vi "Stop.vi"(8 "Error In":errorcluster, 11 "object in":refnum<class "OWON SDS1022.lvclass">) -> (0 "Error Out":errorcluster, 3 "object out":refnum<class "OWON SDS1022.lvclass">)   [LabVIEW 2023, in "OWON SDS1022.lvlib" / "OWON SDS1022.lvclass"]
uses:
  OWON SDS1022.lvclass
  OWON SDS1022.lvclass/OWON SDS1022.ctl
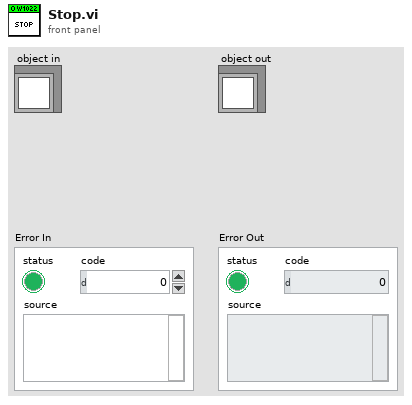
[diagram p1: front panel]
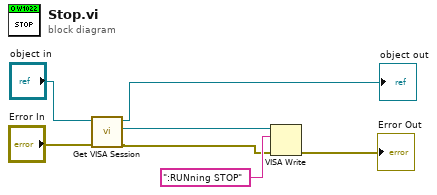
[diagram p0: block diagram]
diagram:
  n1 = call-dynamic "Get VISA Session.vi"("error in"="Error In", "Scope VISA in"="object in") -> ("error out"=w1:errorcluster, "VISA session"=w7:refnum<visa-resource-name>, "Scope VISA out"=→"object out":refnum<class "OWON SDS1022.lvclass">)  [unwired: 7 in]
  n2 = VISA Write(VISA resource name=w7, write buffer=":RUNning STOP", error in (no error)=w1) -> (error out=→"Error Out":errorcluster)  [unwired: 2 out]
